vi "Configure Run VI.vi"(8 "error in (no error)":errorcluster, 11 "JSON string":string) -> (0 "error out":errorcluster, 3 "Run VI Out":refnum<class "Run VI.lvclass">)   [LabVIEW 2014, in "Run VI.lvclass"]
uses:
  Run VI.lvclass
  Shared/Controls/Run VI - STYP.ctl
  Classes/Job/Job.lvclass/Job.ctl
  Run VI.lvclass/Run VI.ctl
  Classes/Job/Write Executor Number.vi
  Write VI Path.vi
  Write Wait Until Done_.vi
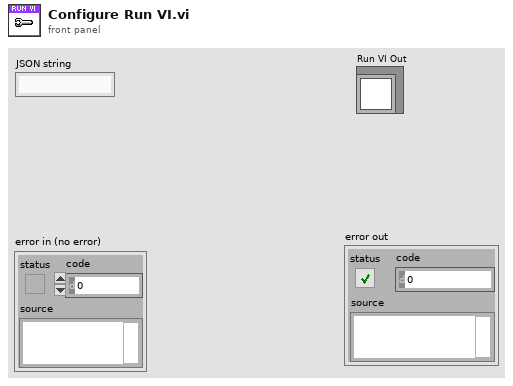
[diagram p1: front panel]
types:
  T1 = typedef "Run VI - STYP.ctl" = cluster{"Executor_Number":string, "VI_Path":string, "Wait_Until_Done":bool}
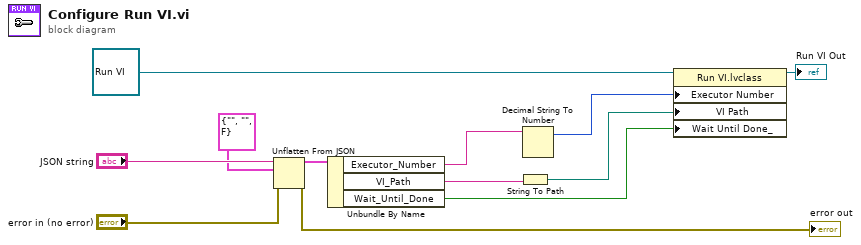
[diagram p0: block diagram]
diagram:
  n1 = Unflatten From JSON(JSON string="JSON string", type and defaults=T1 {"Executor_Number"="", "VI_Path"="", "Wait_Until_Done"=FALSE} ("Run VI"), error in (no error)="error in (no error)") -> (value=w9:T1, error out=→"error out":errorcluster)  [unwired: 4 in]
  n2 = Unbundle By Name(w9) -> ("Executor_Number"=w8:string, "VI_Path"=w5:string, "Wait_Until_Done"=w3:bool)
  n3 = String To Path(string=w5) -> (path=w4:path)
  n4 = Decimal String To Number(string=w8) -> (offset past number=w6:i32)  [unwired: 2 in, 1 out]
  n5 = property class="Run VI.lvclass"(reference=refnum<class "Run VI.lvclass"> refnum ("Run VI.lvclass"), "Executor Number"=w6, "VI Path"=w4, "Wait Until Done_"=w3) -> (reference out=→"Run VI Out":refnum<class "Run VI.lvclass">)  [unwired: 1 in, 1 out]
